vi "Global for awg.vi"() -> ()   [LabVIEW 2024]
panel:
  in  "Cluster":T1={"BW [MHz]"=19.691598360655735, "Taod [us]"=29.10737386804657, "Nzf"=5, "Tpp [us]"=217.72315653298836, "Tdaod [us]"=1357.142857142857, "Tf2 [us]"=2395.569210866753, "Nv"=4.0}
  in  "config":T2={"BW [MHz]"=19.691598360655735, "Taod [us]"=29.10737386804657, "Nzf"=5, "Tpp [us]"=217.72315653298836, "Tdaod [us]"=1357.142857142857, "Tf2 [us]"=2395.569210866753, "Nv"=4.0, "ch1 range"=580.0, "ch2 range"=680.0, "wavel ratio"=0.871, "delay [us]"=-40.0}
  in  "Tex":dbl
  in  "Ny":dbl
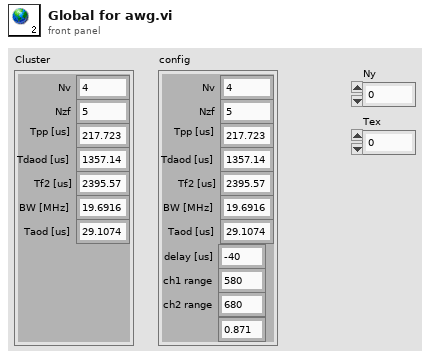
[diagram p1: front panel]
types:
  T1 = cluster{"BW [MHz]":dbl, "Taod [us]":dbl, "Nzf":i32, "Tpp [us]":dbl, "Tdaod [us]":dbl, "Tf2 [us]":dbl, "Nv":dbl}
  T2 = cluster{"BW [MHz]":dbl, "Taod [us]":dbl, "Nzf":i32, "Tpp [us]":dbl, "Tdaod [us]":dbl, "Tf2 [us]":dbl, "Nv":dbl, "ch1 range":dbl, "ch2 range":dbl, "wavel ratio":dbl, "delay [us]":dbl}
diagram:
